vi "Field_from_HP3478A_with_neg.vi"(0 "GPIB Address":string="22") -> (1 "kOe":dbl, 2 "Tesla":dbl, 3 "Oe":dbl)   [LabVIEW 2015]
panel:
  out "Vout":dbl
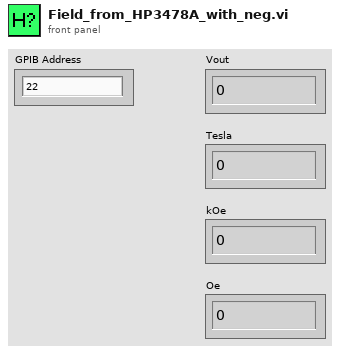
[diagram p1: front panel]
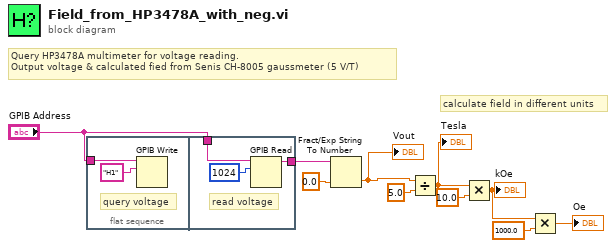
[diagram p0: block diagram]
diagram:
  # "calculate field in different units"
  # "Query HP3478A multimeter for voltage reading.\nOutput voltage & calculated fied from Senis CH-8005 gaussmeter (5 V/T)"
  n1 = flat-sequence {
    tunnel: "GPIB Address" -> [w11]
    tunnel: "GPIB Address" -> [w15]
    tunnel: [w13] -> w7
    frame #0 {
      # "query voltage"
      n2 = GPIB Write(0:w11, 1:"H1" ("data")) -> ()  [unwired: 3 in, 2 out]
    }
    frame #1 {
      # "read voltage"
      n3 = GPIB Read(0:w15, 1:1024 ("byte count")) -> (5:w13:string)  [unwired: 3 in, 2 out]
    }
  }
  n4 = Fract/Exp String To Number(string=w7, default (0 dbl)=0.0 ("default (0 I32)")) -> (number=w1:dbl)  [unwired: 2 in, 1 out]
  "Vout" <- w1
  n5 = Divide(x=w1, y=5.0) -> (x/y=w6:dbl)
  "Tesla" <- w6
  n6 = Multiply(x=w6, y=10.0) -> (x*y=w4:dbl)
  "kOe" <- w4
  n7 = Multiply(x=w4, y=1000.0) -> (x*y=→"Oe":dbl)
